vi "New XML Configuration.vi"(6 "schemaVersion (item12 - 1.2)":i32(ring)=3 items=["Undefined", "Item10", "Item11", "Item12"], 8 "error in":errorcluster, 11 "name(CoreName)":string="CoreName") -> (0 "error out":errorcluster, 3 "xml ref out":refnum<k24>)   [LabVIEW 2020, in "Ballard_1553_Hardware_ni.lvlib"]
uses:
  Ballard_1553_Hardware_ni.lvlib
  C:/Users/Administrator/Desktop/GIT/Ballard-MIL-STD-1553-Custom-Device/Source/System Explorer/SubVIs/Parse XML Ballard/1.2/BTIXML_SerDes.dll
  Ballard-MIL-STD-1553-Custom-Device/Source/System Explorer/SubVIs/Parse XML Ballard/1.2/BTIXML_SerDes.dll
  _typedefs/idManager_action.ctl
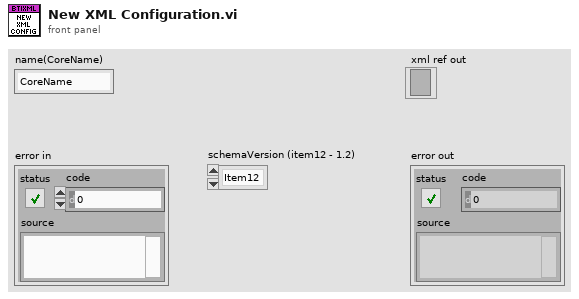
[diagram p1: front panel]
types:
  T1 = typedef "Ballard_1553_Hardware_ni.lvlib/idManager_action.ctl" = enum16{"Increment", "Get", "Set"}
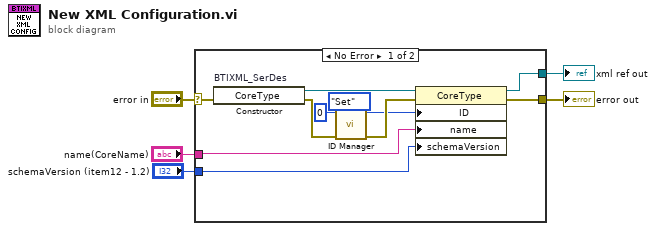
[diagram p0: block diagram]
diagram:
  n1 = case shown="No Error" "error in" {
    selector: "error in" -> [w15 w17]
    tunnel: [w14 w17] -> w4
    tunnel: [w13 _] -> w3
    tunnel: "name(CoreName)" -> [w12 _]
    tunnel: "schemaVersion (item12 - 1.2)" -> [w11 _]
    frame No Error {
      n2 = constructor on="BTIXML_SerDes" class="CoreType"(error in=w15) -> (reference out=w16:refnum<k24>, error out=w10:errorcluster)  [unwired: 2 in, 1 out]
      n3 = call "ID Manager.vi"("action (Increment)"=idManager_action."Set", "error in"=w10, "manual ID"=0) -> ("error out"=w9:errorcluster, "ID out"=w8:i32)  [unwired: 7 in]
      n4 = property class="CoreType"(reference=w16, error in=w9, "ID"=w8, "name"=w12, "schemaVersion"=w11) -> (reference out=w13:refnum<k24>, error out=w14:errorcluster)
    }
    frame Error {
    }
  }
  "error out" <- w4
  "xml ref out" <- w3
